vi "MoveBlock.vi"(8 "error in (no error)":errorcluster, 9 "size":i32, 10 "destination (type)":u8[](array[numeric]), 11 "Address (pointer)":u64) -> (0 "error out":errorcluster, 2 "Value":u8[](array[numeric]) format="%x")   [LabVIEW 2020, in "sqlite3.lvlib"]
uses:
  sqlite3.lvlib
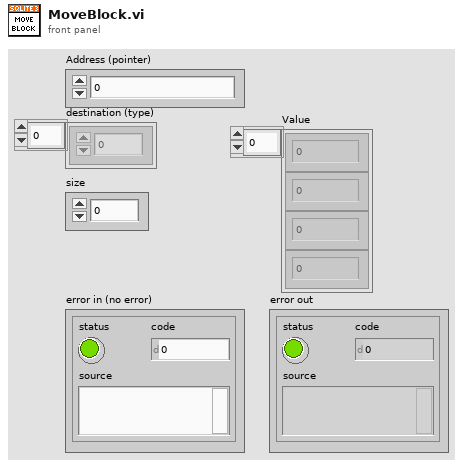
[diagram p1: front panel]
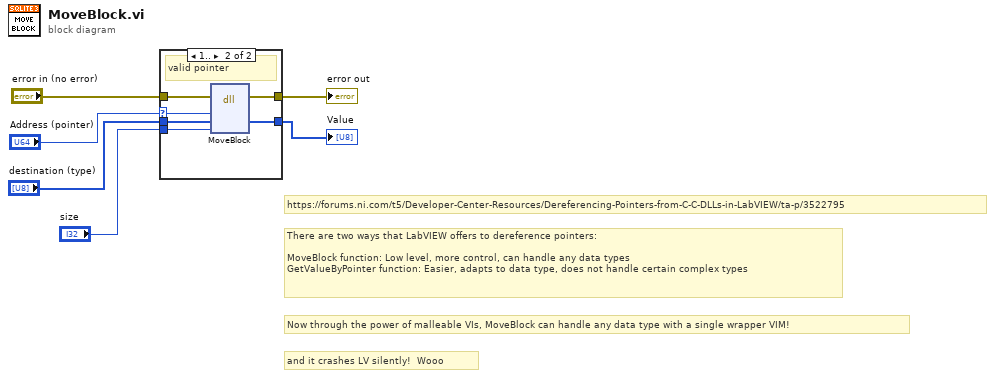
[diagram p0: block diagram]
diagram:
  # "and it crashes LV silently!  Wooo"
  # "Now through the power of malleable VIs, MoveBlock can handle any data type with a single wrapper VIM!"
  # "There are two ways that LabVIEW offers to dereference pointers:\n\nMoveBlock function: Low level, more control, can handle any data types\nGetValueByPointer function: Easier, adapts to data type, does not handle certain complex types"
  # "https://forums.ni.com/t5/Developer-Center-Resources/Dereferencing-Pointers-from-C-C-DLLs-in-LabVIEW/ta-p/3522795"
  n1 = case shown="1.." "Address (pointer)" {
    selector: "Address (pointer)" -> [_ w12]
    tunnel: "error in (no error)" -> [w7 w13]
    tunnel: "size" -> [_ w11]
    tunnel: [w7 w10] -> w3
    tunnel: "destination (type)" -> [_ w9]
    tunnel: [_ w8] -> w1
    frame 0, Default {
      # "null pointer"
    }
    frame 1.. {
      # "valid pointer"
      n2 = dll-call lib="LabVIEW" fn="MoveBlock"(error in=w13, "address"=w12, "destination"=w9, "size"=w11) -> (error out=w10:errorcluster, "destination"=w8:u8[])  [unwired: 5 in, 1 out]
    }
  }
  "error out" <- w3
  "Value" <- w1
